vi "WLAN Configure OFDM ModAcc.vi"(0 "Instrument Handle In":refnum<k21>, 1 "Selector String":string, 5 "OFDM ModAcc Configuration":T1={"Acquisition Length (s)"=0.0, "Averaging Enabled"=0, "Averaging Count"=10, "Optimize Dynamic Range for EVM Enabled"=1, "Optimize Dynamic Range for EVM Margin (dB)"=0.0, "Measurement Offset (sym)"=0, "Maximum Measurement Length (sym)"=16} {"Optimize Dynamic Range for EVM Margin (dB)" format="%.2f"; "Optimize Dynamic Range for EVM Enabled" items=["False", "True"]; "Averaging Enabled" items=["False", "True"]; "Acquisition Length (s)" format="%.3p"}, 11 "error in (no error)":errorcluster) -> (4 "Instrument Handle Out":refnum<k21>, 15 "error out":errorcluster)   [LabVIEW 2016, in "RFmxWLAN.lvlib"]
doc: "Configures common settings for the OFDM ModAcc measurement and selects the measurement."
uses:
  RFmxWLAN.lvlib
  Typedefs/WLAN OFDM ModAcc Configuration.ctl
  <vilib>/RFmx/WLAN/mx/RFmxWLAN.llb/RFmxWLAN Select Measurement (Single).vi
  <resource>/objmgr/RFmxWLAN.rc
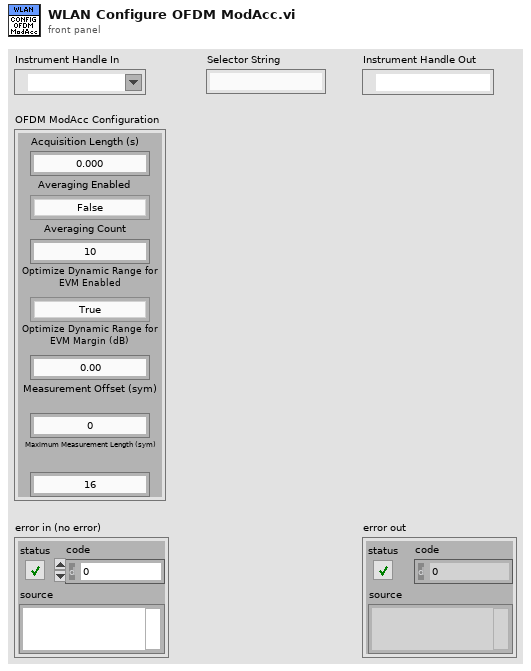
[diagram p1: front panel]
types:
  T1 = typedef "RFmxWLAN.lvlib/WLAN OFDM ModAcc Configuration.ctl" = cluster{"Acquisition Length (s)":dbl, "Averaging Enabled":i32, "Averaging Count":i32, "Optimize Dynamic Range for EVM Enabled":i32, "Optimize Dynamic Range for EVM Margin (dB)":dbl, "Measurement Offset (sym)":i32, "Maximum Measurement Length (sym)":i32}
  T2 = enum16{"TXP", "PowerRamp", "DSSSModAcc", "OFDMModAcc", "SEM"}
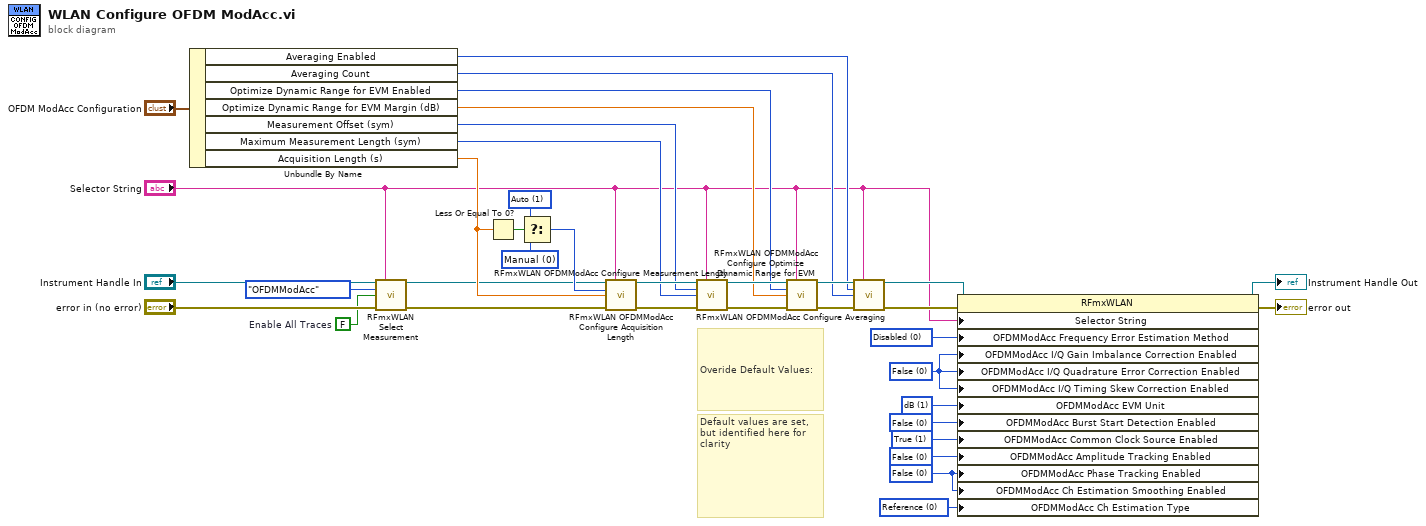
[diagram p0: block diagram]
diagram:
  w1 = 0 items=["Reference", "Reference and Data"] ("OFDMModAcc Ch Estimation Type")
  w2 = FALSE  # Enable All Traces
  w19 = 1 items=["Manual", "Auto"] ("Acquisition Length Mode")
  w17 = 0 items=["Manual", "Auto"] ("Acquisition Length Mode")
  w31 = 0 items=["False", "True"] ("OFDMModAcc Amplitude Tracking Enabled")
  w32 = 0 items=["False", "True"] ("OFDMModAcc Amplitude Tracking Enabled")
  w33 = 1 items=["False", "True"] ("OFDMModAcc Burst Start Detection Enabled")
  w34 = 0 items=["False", "True"] ("OFDMModAcc Burst Start Detection Enabled")
  w35 = 1 items=["Percentage", "dB"] ("OFDMModAcc EVM Unit")
  w36 = 0 items=["False", "True"] ("OFDMModAcc I/Q Quadrature Error Correction Enabled")
  w37 = 0 items=["Disabled", "Initial Preamble", "Preamble", "Preamble and Pilots", "Preamble, Pilots and Data"] ("OFDMModAcc Frequency Error Estimation Method")
  # "Default values are set, but identified here for clarity"
  # "Overide Default Values:"
  n1 = Unbundle By Name("OFDM ModAcc Configuration") -> ("Averaging Enabled"=w10:i32, "Averaging Count"=w11:i32, "Optimize Dynamic Range for EVM Enabled"=w12:i32, "Optimize Dynamic Range for EVM Margin (dB)"=w13:dbl, "Measurement Offset (sym)"=w15:i32, "Maximum Measurement Length (sym)"=w14:i32, "Acquisition Length (s)"=w8:dbl)
  n2 = call-poly <vilib>:"RFmxWLAN Select Measurement.vi"("Instrument Handle In"="Instrument Handle In", "Selector String"="Selector String", "Measurement"=T2."OFDMModAcc", "Enable All Traces"=w2, "error in (no error)"="error in (no error)") -> ("Instrument Handle Out"=w5:refnum<k21>, "error out"=w7:errorcluster)  [unwired: 9 in]
  n3 = Less Or Equal To 0?(x=w8) -> (x <= 0?=w20:bool)
  n4 = Select(t=w19, s=w20, f=w17) -> (s? t:f=w18:i32)
  n5 = call <vilib>:"RFmxWLAN OFDMModAcc Configure Acquisition Length.vi"("Instrument Handle In"=w5, "Selector String"="Selector String", "Acquisition Length Mode"=w18, "Acquisition Length (s)"=w8, "error in (no error)"=w7) -> ("Instrument Handle Out"=w25:refnum<k21>, "error out"=w24:errorcluster)  [unwired: 9 in]
  n6 = call <vilib>:"RFmxWLAN OFDMModAcc Configure Measurement Length.vi"("Instrument Handle In"=w25, "Selector String"="Selector String", "Measurement Offset (symbols)"=w15, "Maximum Measurement Length (symbols)"=w14, "error in (no error)"=w24) -> ("Instrument Handle Out"=w27:refnum<k21>, "error out"=w26:errorcluster)  [unwired: 9 in]
  n7 = call <vilib>:"RFmxWLAN OFDMModAcc Configure Optimize Dynamic Range for EVM.vi"("Instrument Handle In"=w27, "Selector String"="Selector String", "Optimize Dynamic Range for EVM Enabled"=w12, "Optimize Dynamic Range for EVM Margin (dB)"=w13, "error in (no error)"=w26) -> ("Instrument Handle Out"=w23:refnum<k21>, "error out"=w22:errorcluster)  [unwired: 9 in]
  n8 = call <vilib>:"RFmxWLAN OFDMModAcc Configure Averaging.vi"("Instrument Handle In"=w23, "Selector String"="Selector String", "Averaging Enabled"=w10, "Averaging Count"=w11, "error in (no error)"=w22) -> ("Instrument Handle Out"=w9:refnum<k21>, "error out"=w28:errorcluster)  [unwired: 9 in]
  n9 = property class="RFmxWLAN"(reference=w9, error in=w28, "Selector String"="Selector String", "OFDMModAcc Frequency Error Estimation Method"=w37, "OFDMModAcc I/Q Gain Imbalance Correction Enabled"=w36, "OFDMModAcc I/Q Quadrature Error Correction Enabled"=w36, "OFDMModAcc I/Q Timing Skew Correction Enabled"=w36, "OFDMModAcc EVM Unit"=w35, "OFDMModAcc Burst Start Detection Enabled"=w34, "OFDMModAcc Common Clock Source Enabled"=w33, "OFDMModAcc Amplitude Tracking Enabled"=w32, "OFDMModAcc Phase Tracking Enabled"=w31, "OFDMModAcc Ch Estimation Smoothing Enabled"=w31, "OFDMModAcc Ch Estimation Type"=w1) -> (reference out=→"Instrument Handle Out":refnum<k21>, error out=→"error out":errorcluster)
